vi "Add Test Information.vi"(8 "error in (no error)":errorcluster, 10 "Test Information":T1, 11 "ResultProcessor in":refnum<class "ResultProcessor.lvclass">) -> (0 "error out":errorcluster, 3 "ResultProcessor out":refnum<class "ResultProcessor.lvclass">)   [LabVIEW 2015, in "ResultProcessor.lvclass"]
doc: "This VI will add just the test execution data to the report."
uses:
  ResultProcessor.lvclass
  Report Information/Test Information.ctl
  CommandQueueDataType.ctl
  Report Information/Report Information.lvclass
  Result/Result.lvclass
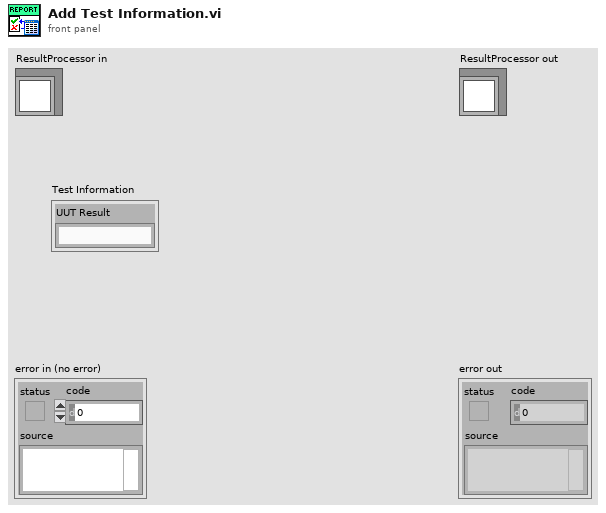
[diagram p1: front panel]
types:
  T1 = typedef "Report Information.lvclass/Test Information.ctl" = cluster{"UUT Result":string}
  T2 = typedef "ResultProcessor.lvclass/CommandQueueDataType.ctl" = cluster{"Command":enum16{"New Report", "Add Result", "Publish Report", "Shutdown", "Add DUT Information", "Add Station Information", "Add Report Information", "Add Test Information"}, "Report Information.lvclass":refnum<class "Report Information.lvclass">, "Result.lvclass":refnum<class "Result.lvclass">}
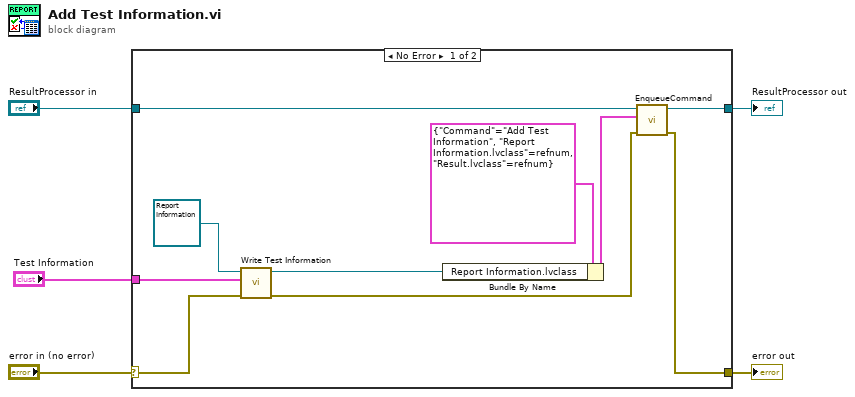
[diagram p0: block diagram]
diagram:
  n1 = case shown="No Error" "error in (no error)" {
    selector: "error in (no error)" -> [w9 w17]
    tunnel: [w13 w17] -> w5
    tunnel: [w14 w16] -> w4
    tunnel: "ResultProcessor in" -> [w15 w16]
    tunnel: "Test Information" -> [w6 _]
    frame No Error {
      n2 = call-dynamic "Write Test Information.vi"("error in (no error)"=w9, "Test Information"=w6, "Report Information in"=refnum<class "Report Information.lvclass"> refnum ("Report Information.lvclass")) -> ("error out"=w8:errorcluster, "Report Information out"=w7:refnum<class "Report Information.lvclass">)  [unwired: 7 in]
      n3 = Bundle By Name(cluster=T2 {"Command"=enum."Add Test Information", "Report Information.lvclass"=refnum, "Result.lvclass"=refnum} ("element"), "Report Information.lvclass"=w7) -> (w11:T2)
      n4 = call "EnqueueCommand.vi"("error in (no error)"=w8, "element"=w11, "ResultProcessor in"=w15) -> ("error out"=w13:errorcluster, "ResultProcessor out"=w14:refnum<class "ResultProcessor.lvclass">)  [unwired: 7 in]
    }
    frame Error {
    }
  }
  "error out" <- w5
  "ResultProcessor out" <- w4
